vi "Start Log File.vi"(8 "error in (no error)":errorcluster, 11 "CLILogger in":refnum<class "CLILogger.lvclass">) -> (0 "error out":errorcluster, 3 "CLILogger out":refnum<class "CLILogger.lvclass">)   [LabVIEW 2020, in "GPackTools.lvlib" / "CLILogger.lvclass"]
uses:
  CLILogger.lvclass
  CLILogger.lvclass/CLILogger.ctl
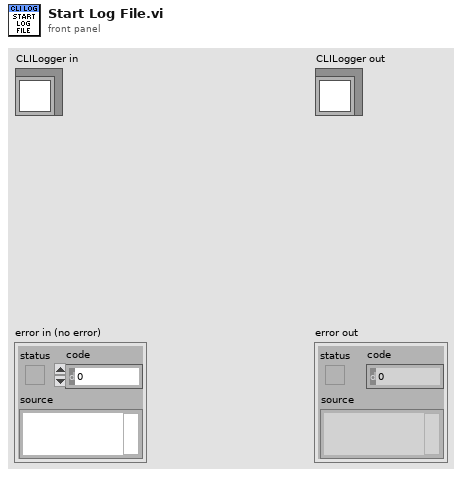
[diagram p1: front panel]
types:
  T1 = enum16{"open", "replace", "create", "open or create", "replace or create", "replace or create with confirmation"}
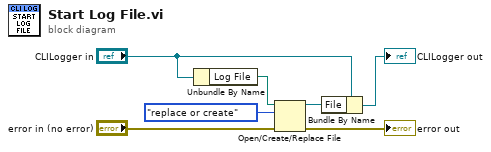
[diagram p0: block diagram]
diagram:
  n1 = Unbundle By Name("CLILogger in") -> ("Log File"=w6:path)
  n2 = Open/Create/Replace File(file path (use dialog)=w6, error in="error in (no error)", operation (0:open)=T1."replace or create") -> (refnum out=w1:refnum<file>, error out=→"error out":errorcluster)  [unwired: 3 in, 1 out]
  n3 = Bundle By Name(cluster="CLILogger in", "File"=w1) -> (→"CLILogger out":refnum<class "CLILogger.lvclass">)
